vi "Vacuum Level Test.vi"(7 "FP":T2, 8 "Results":T1[](array[typedef]), 10 "VacPass":bool[](array[boolean]), 11 "Cart Array":bool[](array[boolean])) -> (1 "Error String":string, 3 "Pass/Fail Array":bool[](array[boolean]))   [LabVIEW 2018]
uses:
  Main Refs.ctl
  Hardware/Tecan/Pump Config.ctl
  Vacuum Specs.ctl
  Cartridges.ctl
  Cartridge Status.ctl
  Commands.ctl
  Lib/Time/Wells.ctl
  Lib/Time/Bottles.ctl
  Process State.ctl
  Vacuum Test.ctl
  Vacuum Output.ctl
  Update Single Cart.ctl
panel:
  # "Tecan Pump"
  # "Vacuum"
  # "General"
  # "Protocol"
  # "Zaber"
  # "NFC Reader 1"
  # "NFC  Reader 2"
  # "NFC Reader 3"
  # "NFC Reader 4"
  # "System"
  # "Cartridge Utitlies"
  # "Wells"
  # "times"
  # "from"
  # "State Machine"
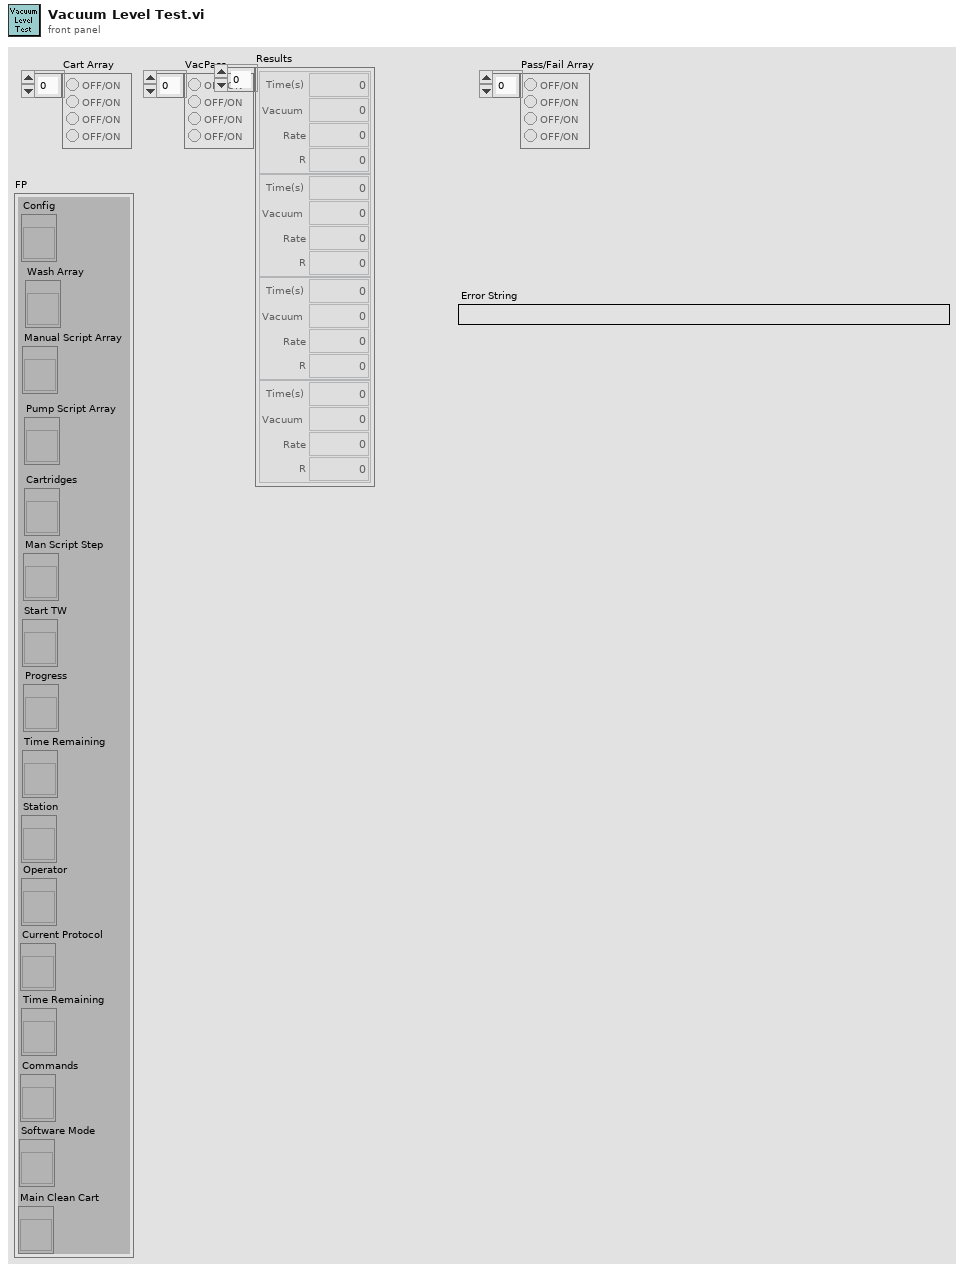
[diagram p1: front panel]
types:
  T1 = typedef "Vacuum Output.ctl" = cluster{"Time(s)":dbl, "Vacuum":dbl, "Rate":dbl, "R":dbl}
  T2 = typedef "Main Refs.ctl" = cluster{"Config":refnum<vi>, "Wash Array":refnum<vi>, "Manual Script Array":refnum<vi>, "Pump Script Array":refnum<vi>, "Cartridges":refnum<vi>, "Man Script Step":refnum<vi>, "Start TW":refnum<vi>, "Progress":refnum<vi>, "Time Remaining":refnum<vi>, "Station":refnum<vi>, "Operator":refnum<vi>, "Current Protocol":refnum<vi>, "Time Remaining":refnum<vi>, "Commands":refnum<vi>, "Software Mode":refnum<vi>, "Main Clean Cart":refnum<vi>}
  T3 = typedef "Update Single Cart.ctl" = enum16{"Cart Status", "Cart Reagent"}
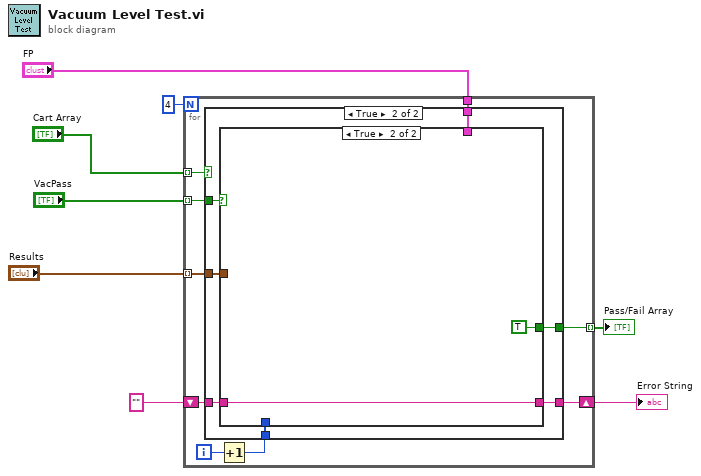
[diagram p0: block diagram]
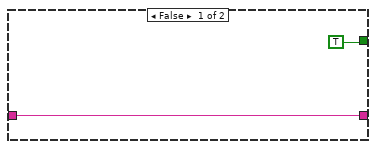
[diagram p2: hidden frame]
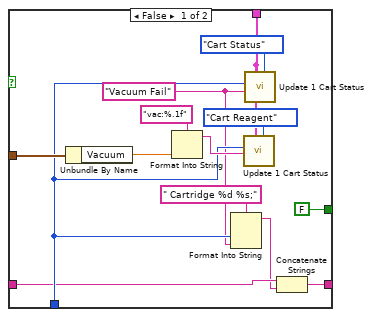
[diagram p3: hidden frame]
diagram:
  n1 = for {
    N: 4 -> [_]
    tunnel: "VacPass" -> [w17] mode=indexing
    tunnel: "Cart Array" -> [w16] mode=indexing
    tunnel: "FP" -> [w15]
    tunnel: "Results" -> [w13] mode=indexing
    shift-right: [w12] -> w7
    shift-left: "" ("String") -> [w11]
    tunnel: [w9] -> w1 mode=indexing
    i -> [w14]
    n2 = Increment(x=w14) -> (x+1=w10:i32)
    n3 = case shown="True" w16 {
      tunnel: w17 -> [_ w24]
      tunnel: w15 -> [_ w26]
      tunnel: w10 -> [_ w25]
      tunnel: w13 -> [_ w23]
      tunnel: w11 -> [w19 w22]
      tunnel: [w19 w21] -> w12
      tunnel: [TRUE w20] -> w9
      frame False {
      }
      frame True {
        n4 = case shown="True" w24 {
          tunnel: w26 -> [w35 _]
          tunnel: w25 -> [w33 _]
          tunnel: w23 -> [w34 _]
          tunnel: w22 -> [w30 w42]
          tunnel: [w28 w42] -> w21
          tunnel: [FALSE TRUE] -> w20
          frame False {
            w32 = "Vacuum Fail" ("String")
            n5 = Unbundle By Name(w34) -> ("Vacuum"=w39:dbl)
            n6 = Format Into String(format string="vac:%.1f", w39) -> (resulting string=w36:string)  [unwired: 2 in, 1 out]
            n7 = Format Into String(format string=" Cartridge %d %s;", w33, w32) -> (resulting string=w29:string)  [unwired: 2 in, 1 out]
            n8 = call "Update 1 Cart Status.vi"("Selection"=Update_Single_Cart."Cart Reagent", "FP"=w35, "String"=w36, "Cartridge"=w33) -> ()  [unwired: 7 in, 1 out]
            n9 = call "Update 1 Cart Status.vi"("Selection"=Update_Single_Cart."Cart Status", "FP"=w35, "String"=w32, "Cartridge"=w33) -> ()  [unwired: 7 in, 1 out]
            n10 = Concatenate Strings(w30, w29) -> (w28:string)
          }
          frame True {
          }
        }
      }
    }
  }
  "Error String" <- w7
  "Pass/Fail Array" <- w1
